vi "ExampleRestartableWriter.vi"() -> ()   [LabVIEW 2011]
uses:
  0x2 Typedefs/RIO-OCU update controls.ctl
  2-Think/2 Typedefs/generalized sensor status.ctl
  2-Think/2 Typedefs/indicator LED.ctl
  2-Think/2 Typedefs/generalized actuator status.ctl
  2-Think/2 Typedefs/Which Boat.ctl
  2-Think/2 Typedefs/robot velocity.ctl
  2-Think/2 Typedefs/UTM Location.ctl
  2-Think/2 Typedefs/heading.ctl
  2-Think/2 Typedefs/rate of turn.ctl
  2-Think/2 Typedefs/pitch and roll.ctl
  2-Think/2 Typedefs/apparent wind.ctl
  2-Think/2 Typedefs/apparent wind speed.ctl
  2-Think/2 Typedefs/apparent wind direction.ctl
  2-Think/2 Typedefs/Velocity.ctl
  2-Think/2 Typedefs/absolute wind direction.ctl
  2-Think/2 Typedefs/absolute wind speed.ctl
  2-Think/2 Typedefs/absolute water current vector.ctl
  2-Think/2 Typedefs/rudder angle.ctl
  2-Think/2 Typedefs/sail setpt.ctl
  0x2 Typedefs/manual override.ctl
  2-Think/2 Typedefs/setpoints to boat.ctl
  0x2 Typedefs/Waypoints List.ctl
  0x2 Typedefs/ocuWaypoint.ctl
  0x2 Typedefs/waypointTypes.ctl
  0x2 Typedefs/Current Waypoint.ctl
  2-Think/2 Globals/2 Global.vi
  Writer/NetworkStreamWriter.lvclass
panel:
  out "Connected?":bool
  in  "Monitored Items from RIO":T1 {"Robot Pitch/Roll"."Roll" format="%05.1f"; "Robot Pitch/Roll"."Pitch" format="%05.1f"; "Robot\nRate of Turn" format="%05.1f"; "Robot\nHeading" format="%05.1f"}
  out "Current iteration":i32
  in  "stop":bool
  # "How Am I?"
  # "Where Am I?"
  # "Path Planning"
  # "From Planning Functions"
  # "(this is not a cluster because subitems\nare generated in parallel code)"
  # "What's Around Me?"
  # "As Measured"
  # "As Measured"
  # "Loop Rates"
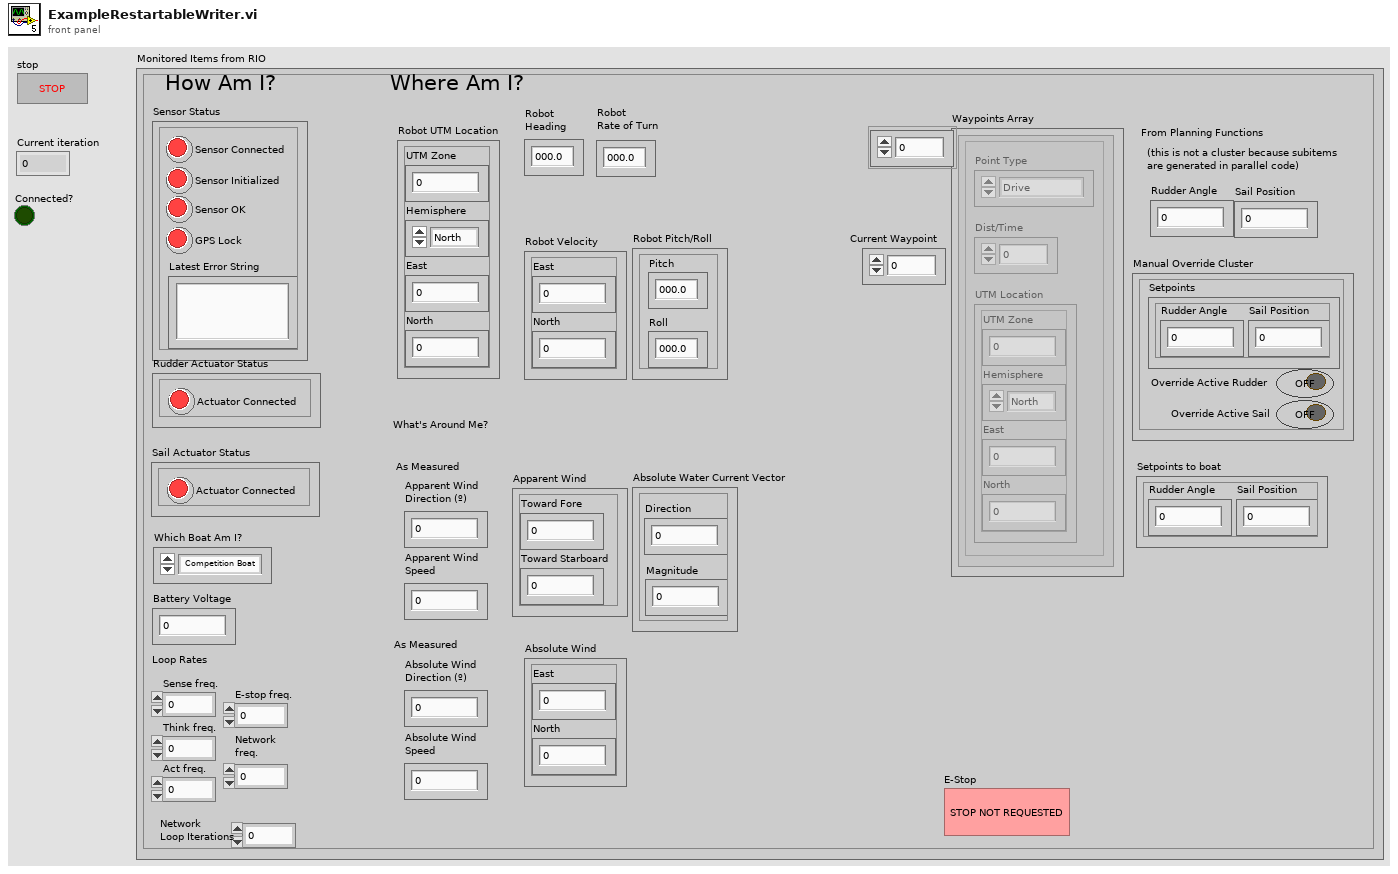
[diagram p1: front panel]
types:
  T1 = typedef "RIO-OCU update controls.ctl" = cluster{"Sensor Status":T2, "Battery Voltage":dbl, "Rudder Actuator Status":T4, "Sail Actuator Status":T4, "Which Boat Am I?":T5, "Robot Velocity":T6, "Robot UTM Location":T7, "Robot\nHeading ":T8, "Robot\nRate of Turn":T9, "Robot Pitch/Roll":T10, "Apparent Wind":T11, "Apparent Wind\nSpeed":T12, "Apparent Wind\nDirection (º)":T13, "Absolute Wind":T14, "Absolute Wind\nDirection (º)":T15, "Absolute Wind\nSpeed":T16, "Absolute Water Current Vector":T17, "Rudder Angle":T18, "Sail Position":T19, "Manual Override Cluster":T20, "Setpoints to boat":T21, "Waypoints Array":T22, "Current Waypoint":T25, "Think freq.":dbl, "Sense freq.":dbl, "Act freq.":dbl, "E-stop freq.":dbl, "Network \nfreq.":dbl, "Network \nLoop Iterations":i64, "E-Stop":bool}
  T2 = typedef "generalized sensor status.ctl" = cluster{"Sensor Connected":T3, "Sensor Initialized":T3, "Sensor OK":T3, "Latest Error String":string, "GPS Lock":T3}
  T3 = typedef "indicator LED.ctl" = bool
  T4 = typedef "generalized actuator status.ctl" = cluster{"Actuator Connected":T3}
  T5 = typedef "Which Boat.ctl" = enum16{"Competition Boat", "Small RC", "Simulation"}
  T6 = typedef "robot velocity.ctl" = cluster{"East":dbl, "North":dbl}
  T7 = typedef "UTM Location.ctl" = cluster{"UTM Zone":dbl, "Hemisphere":enum16{"North", "South"}, "East":dbl, "North":dbl}
  T8 = typedef "heading.ctl" = dbl
  T9 = typedef "rate of turn.ctl" = dbl
  T10 = typedef "pitch and roll.ctl" = cluster{"Pitch":dbl, "Roll":dbl}
  T11 = typedef "apparent wind.ctl" = cluster{"Toward Fore":dbl, "Toward Starboard":dbl}
  T12 = typedef "apparent wind speed.ctl" = dbl
  T13 = typedef "apparent wind direction.ctl" = dbl
  T14 = typedef "Velocity.ctl" = cluster{"East":dbl, "North":dbl}
  T15 = typedef "absolute wind direction.ctl" = dbl
  T16 = typedef "absolute wind speed.ctl" = dbl
  T17 = typedef "absolute water current vector.ctl" = cluster{"Direction":T13, "Magnitude":T13}
  T18 = typedef "rudder angle.ctl" = dbl
  T19 = typedef "sail setpt.ctl" = dbl
  T20 = typedef "manual override.ctl" = cluster{"Override Active Rudder":bool, "Setpoints":T21, "Override Active Sail":bool}
  T21 = typedef "setpoints to boat.ctl" = cluster{"Sail Position":T19, "Rudder Angle":T18}
  T22 = typedef "Waypoints List.ctl" = T23[]
  T23 = typedef "ocuWaypoint.ctl" = cluster{"Point Type":T24, "Dist/Time":dbl, "UTM Location":T7}
  T24 = typedef "waypointTypes.ctl" = enum16{"Drive", "Round Port", "Round Starboard", "Stay"}
  T25 = typedef "Current Waypoint.ctl" = i32
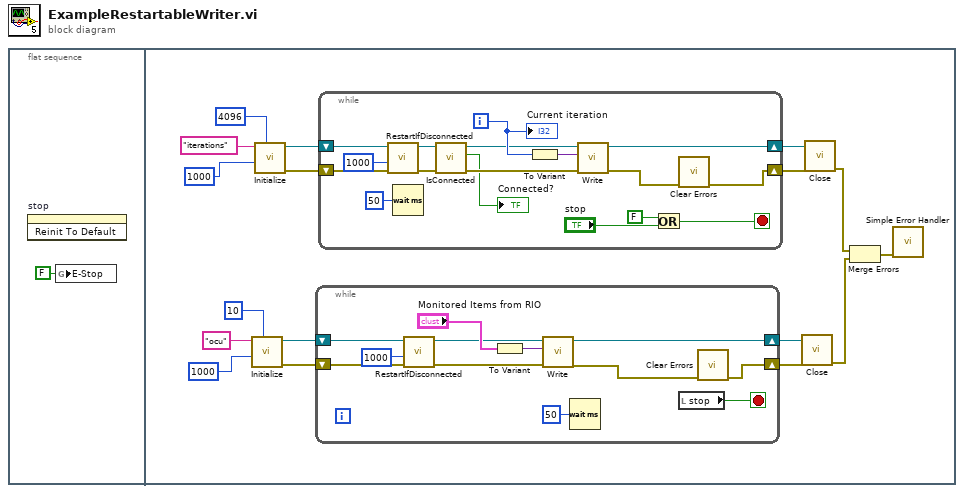
[diagram p0: block diagram]
diagram:
  n1 = flat-sequence {
    frame #0 {
      n2 = invoke on="stop" class="Bool (strict)" method="Reinit To Default"() -> ()  [unwired: 3 in, 3 out]
      n3 = global write "2 Global.vi" "E-Stop"(FALSE ("E-Stop")) -> ()
    }
    frame #1 {
      n4 = call "Initialize.vi"("writer buffer size"=10, "connection timeout"=1000, "writer name"="ocu") -> ("error out"=w10:errorcluster, "NetworkStreamWriter out"=w9:refnum<class "NetworkStreamWriter.lvclass">)  [unwired: 6 in, 1 out]
      n5 = call "Initialize.vi"("writer buffer size"=4096, "connection timeout"=1000, "writer name"="iterations") -> ("error out"=w17:errorcluster, "NetworkStreamWriter out"=w18:refnum<class "NetworkStreamWriter.lvclass">)  [unwired: 6 in, 1 out]
      n6 = while {
        shift-right: [w25] -> w13
        shift-left: w10 -> [w23]
        shift-right: [w20] -> w12
        shift-left: w9 -> [w24]
        stop <- w27 stop-if-true
        n7 = call "RestartIfDisconnected.vi"("error in (no error)"=w23, "connection timeout"=1000, "NetworkStreamWriter in"=w24) -> ("error out"=w21:errorcluster, "NetworkStreamWriter out"=w22:refnum<class "NetworkStreamWriter.lvclass">)  [unwired: 7 in]
        n8 = To Variant(anything="Monitored Items from RIO") -> (Variant=w30:variant)
        n9 = call "Write.vi"("error in (no error)"=w21, "element"=w30, "NetworkStreamWriter in"=w22) -> ("error out"=w19:errorcluster, "NetworkStreamWriter out"=w20:refnum<class "NetworkStreamWriter.lvclass">)  [unwired: 6 in, 1 out]
        n10 = Wait (ms)(milliseconds to wait=u32 50) -> ()  [unwired: 1 out]
        n11 = local read "stop"() -> (w27:bool)
        n12 = call <vilib>:"Clear Errors.vi"("error in (no error)"=w19) -> ("error out"=w25:errorcluster)  [unwired: 6 in]
      }
      n13 = while {
        shift-right: [w37] -> w14
        shift-left: w17 -> [w35]
        shift-right: [w32] -> w15
        shift-left: w18 -> [w36]
        i -> [w47]
        stop <- w43 stop-if-true
        n14 = call "RestartIfDisconnected.vi"("error in (no error)"=w35, "connection timeout"=1000, "NetworkStreamWriter in"=w36) -> ("error out"=w33:errorcluster, "NetworkStreamWriter out"=w34:refnum<class "NetworkStreamWriter.lvclass">)  [unwired: 7 in]
        n15 = Wait (ms)(milliseconds to wait=u32 50) -> ()  [unwired: 1 out]
        n16 = call "IsConnected.vi"("error in (no error)"=w33, "NetworkStreamWriter in"=w34) -> ("error out"=w41:errorcluster, "Connected?"=→"Connected?":bool, "NetworkStreamWriter out"=w42:refnum<class "NetworkStreamWriter.lvclass">)  [unwired: 7 in]
        n17 = To Variant(anything=w47) -> (Variant=w46:variant)
        n18 = call "Write.vi"("error in (no error)"=w41, "element"=w46, "NetworkStreamWriter in"=w42) -> ("error out"=w31:errorcluster, "NetworkStreamWriter out"=w32:refnum<class "NetworkStreamWriter.lvclass">)  [unwired: 6 in, 1 out]
        n19 = Or(x=FALSE, y="stop") -> (x .or. y?=w43:bool)
        n20 = call <vilib>:"Clear Errors.vi"("error in (no error)"=w31) -> ("error out"=w37:errorcluster)  [unwired: 6 in]
        "Current iteration" <- w47
      }
      n21 = call "Close.vi"("error in (no error)"=w13, "NetworkStreamWriter in"=w12) -> ("error out"=w7:errorcluster)  [unwired: 8 in, 1 out]
      n22 = call "Close.vi"("error in (no error)"=w14, "NetworkStreamWriter in"=w15) -> ("error out"=w8:errorcluster)  [unwired: 8 in, 1 out]
      n23 = Merge Errors(w8, w7) -> (w6:errorcluster)
      n24 = call <vilib>:"Simple Error Handler.vi"("error in (no error)"=w6) -> ()  [unwired: 4 in, 5 out]
    }
  }
